vi "configuration UI.vi"() -> ()   [LabVIEW 2015, in "UI Reference editor node.lvclass"]
uses:
  UI Reference editor node.lvclass
  <vilib>/NI/Configuration Framework/Node/NodeRef.ctl
  <vilib>/NI/Configuration Framework/Node/NISE_CEF_Node.lvclass
  <vilib>/NI/AMC/Message Queue.ctl
  <vilib>/NI/AMC/Message.ctl
  <vilib>/NI/Tools/Keyed Array/KeyedArray.ctl
  <vilib>/NI/Configuration Framework/Node/UserEventRef.ctl
  <vilib>/NI/Configuration Framework/Controls/EventCluster.ctl
  <vilib>/NI/DCAF UI Toolkit/Controls/Configure.ctl
  <vilib>/NI/DCAF UI Toolkit/Controls/Add.ctl
  <vilib>/NI/DCAF UI Toolkit/Controls/Remove.ctl
  module/configuration/UI Reference configuration.lvclass
  <vilib>/Utility/miscctls.llb/LVPositionTypeDef.ctl
  <vilib>/NI/Module Execution Interface/Engine Configuration/engine configuration.lvclass
  <vilib>/NI/DCAF/Tag Editor Core/Configuration Editor/Classes/Engine Parent/Engine Parent Editor Node.lvclass
  <vilib>/NI/Tag Bus/tag/tag descriptor.lvclass
  <vilib>/NI/Tag Bus/tag/Data Type.ctl
  <vilib>/NI/Tag Bus/tag/tag descriptor.lvclass/tag descriptor.ctl
  module/configuration/UI Reference configuration.lvclass/UI Reference configuration.ctl
  UI Reference editor node.lvclass/UI Reference editor node.ctl
  <vilib>/NI/Tag Bus/tag/write tag name.vi
  <vilib>/NI/Tag Bus/tag/write data type.vi
  module/configuration/Read VI name.vi
  <vilib>/NI/DCAF/Tag Editor Core/Configuration Editor/Classes/Module editor node/Read Module Configuration.vi
  <vilib>/NI/Configuration Framework/serializable configuration/NISE_CEF_serializable configuration.lvclass
  <vilib>/NI/Tag Bus Module Framework/module configuration/TBM module configuration.lvclass
  <vilib>/NI/Configuration Framework/NISE_CEF_TreeControl.lvlib
  <vilib>/NI/DCAF/Tag Editor Core/Configuration Editor/Classes/Module editor node/module editor node.lvclass
  <vilib>/NI/DCAF UI Toolkit/Controls/DCAF UI Elements.lvlib
  <vilib>/NI/Tools/Keyed Array/Tools_KeyedArray.lvlib
  <vilib>/NI/AMC/AMC.lvlib
panel:
  in  "Top Level Tab Control":enum32{"UI Configuration"}(tab)
  in  "channel":i32(listbox)
  out "UI to Load":string
  in  "browse":bool
  in  "autogen":bool
  in  "Add Button":T1
  in  "Remove Button":T2
  in  "settings":T3
  in  "hidden_Add":bool
  in  "hidden_settings":bool
  in  "hidden_remove":bool
  in  "user event":T4
  in  "main queue":T5
  in  "node ref":T6
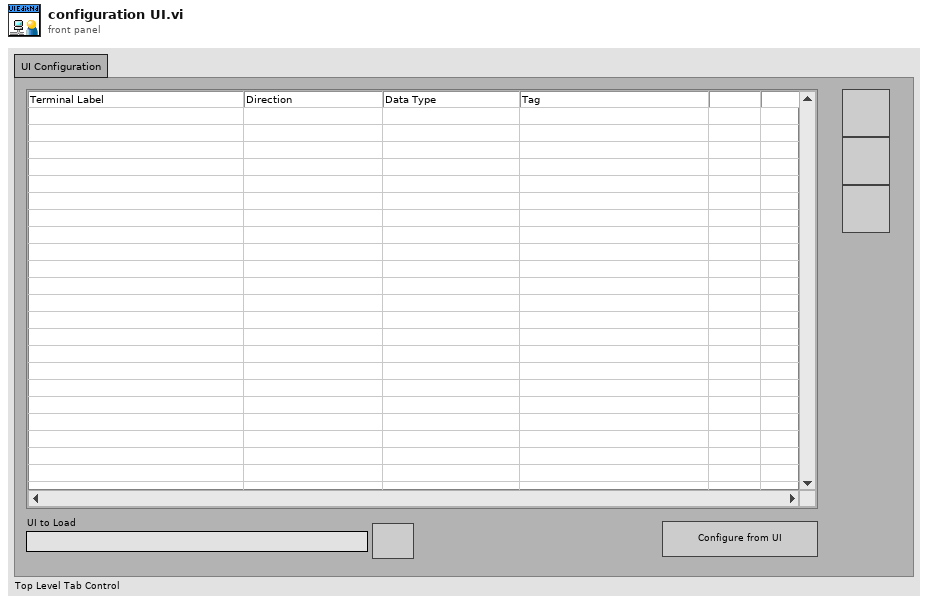
[diagram p1: front panel]
types:
  T1 = typedef "DCAF UI Elements.lvlib/Add.ctl" = bool
  T2 = typedef "DCAF UI Elements.lvlib/Remove.ctl" = bool
  T3 = typedef "DCAF UI Elements.lvlib/Configure.ctl" = bool
  T4 = typedef "NISE_CEF_Node.lvclass/UserEventRef.ctl" = refnum<user-event>
  T5 = typedef "AMC.lvlib/Message Queue.ctl" = refnum<queue>
  T6 = typedef "NISE_CEF_Node.lvclass/NodeRef.ctl" = refnum<data-value>
  T7 = typedef "LVPositionTypeDef.ctl" = cluster{"Left":i32, "Top":i32}
  T8 = typedef "NISE_CEF_TreeControl.lvlib/EventCluster.ctl" = cluster{"command":string, "data":string}
  T9 = typedef "tag bus.lvlib/tag descriptor.lvclass/Data Type.ctl" = enum16{"Double", "Single", "I64", "I32", "I16", "I8", "U64", "U32", "U16", "U8", "Boolean", "String", "Array of Double", "Array of Single", "Array of I64", "Array of I32", "Array of I16", "Array of I8", "Array of U64", "Array of U32", "Array of U16", "Array of U8", "Array of Boolean", "Array of String"}
  T10 = typedef "UI Reference editor node.lvclass/table line.ctl" = cluster{"channel":refnum<class "TBM channel.lvclass">, "tag name":string}
  T11 = typedef "LVPoint32TypeDef.ctl" = cluster{"Horizontal":i32, "Vertical":i32}
  T12 = typedef "LVRowAndColumnTypeDef.ctl" = cluster{"Row":i32, "Column":i32}
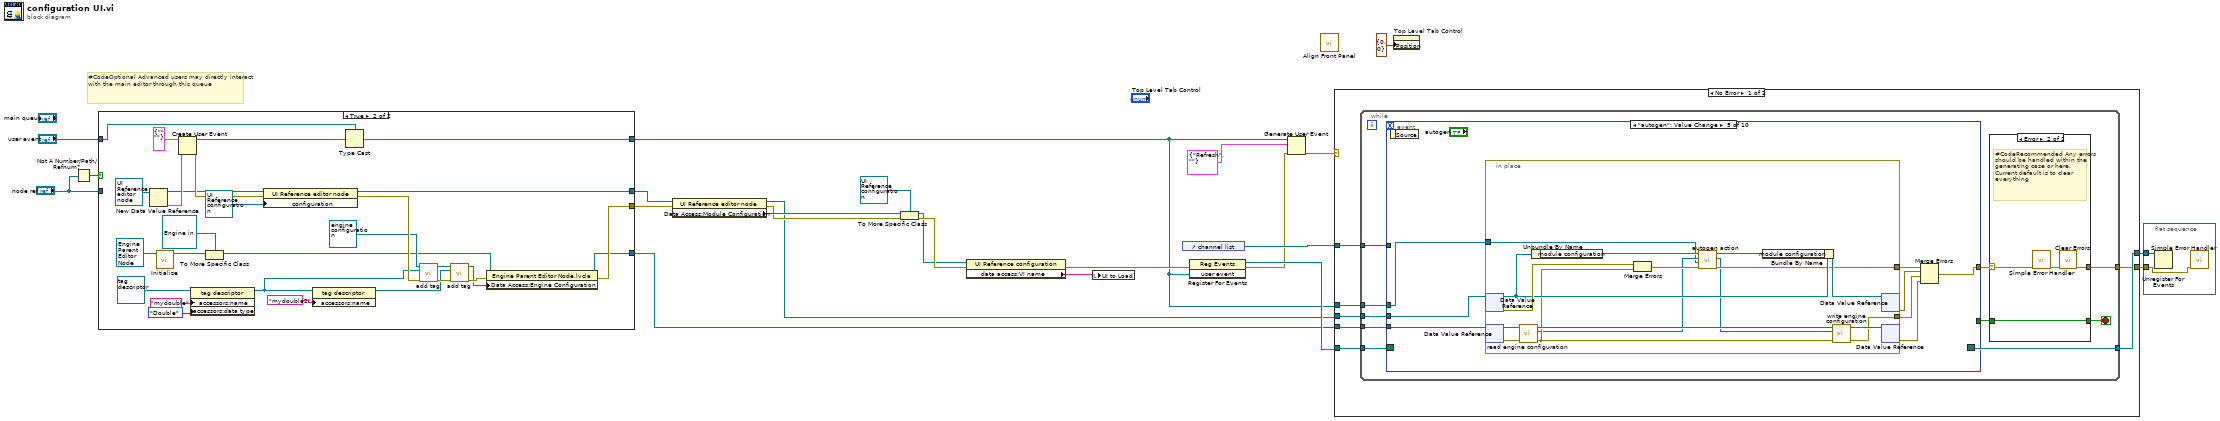
[diagram p0: block diagram]
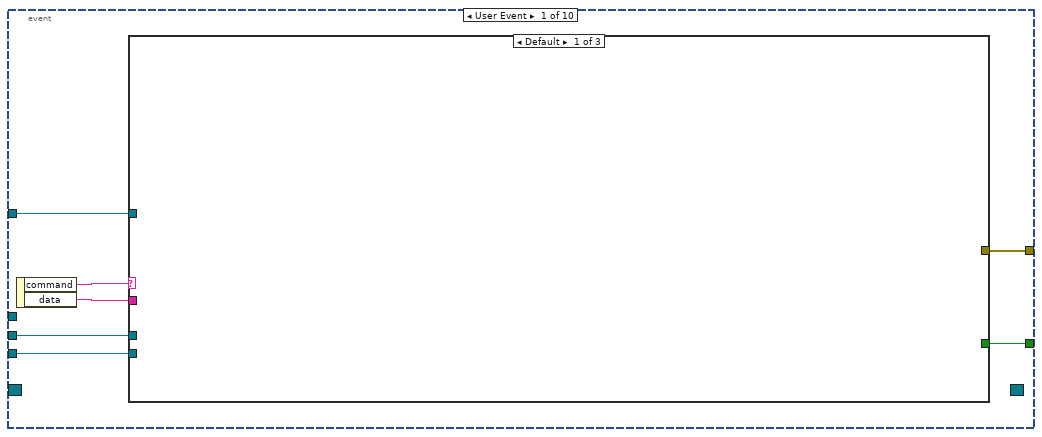
[diagram p3: hidden frame]
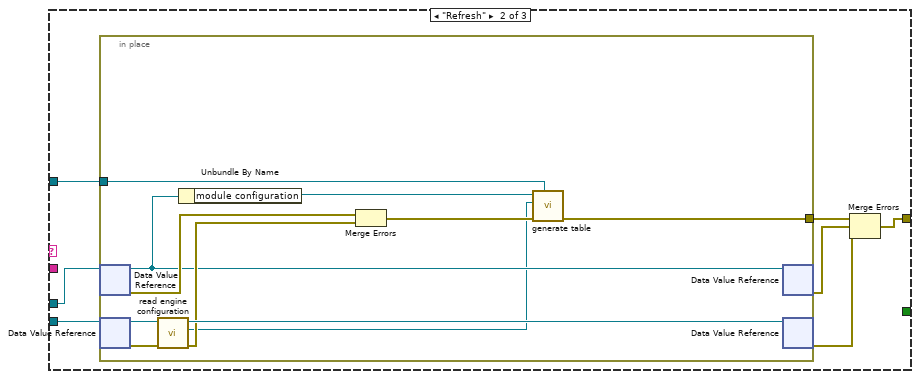
[diagram p4: hidden frame]
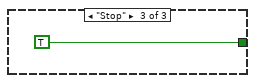
[diagram p5: hidden frame]
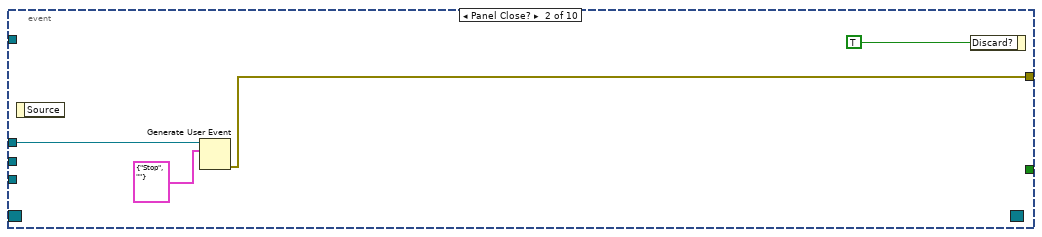
[diagram p6: hidden frame]
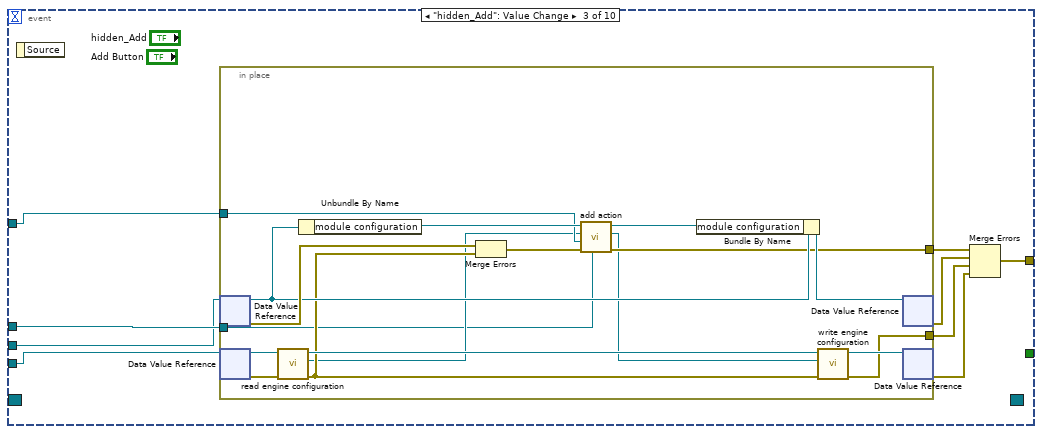
[diagram p7: hidden frame]
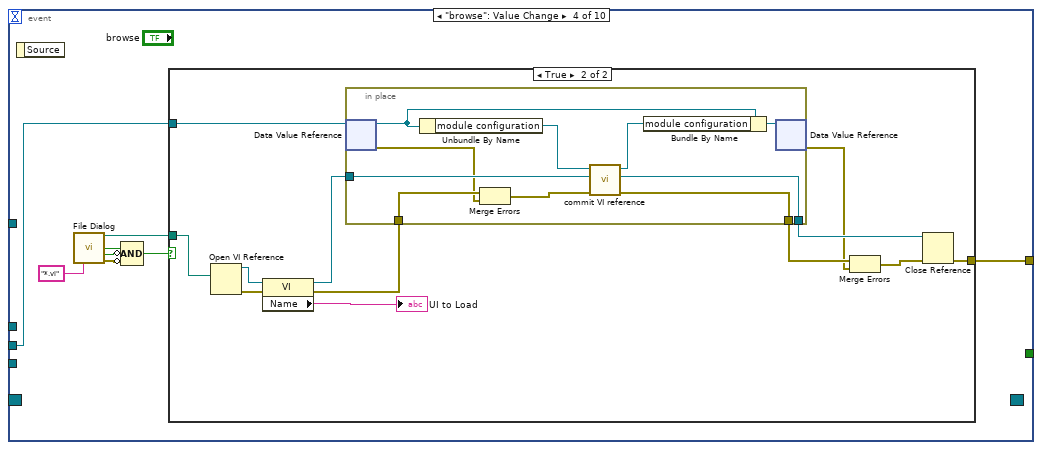
[diagram p8: hidden frame]
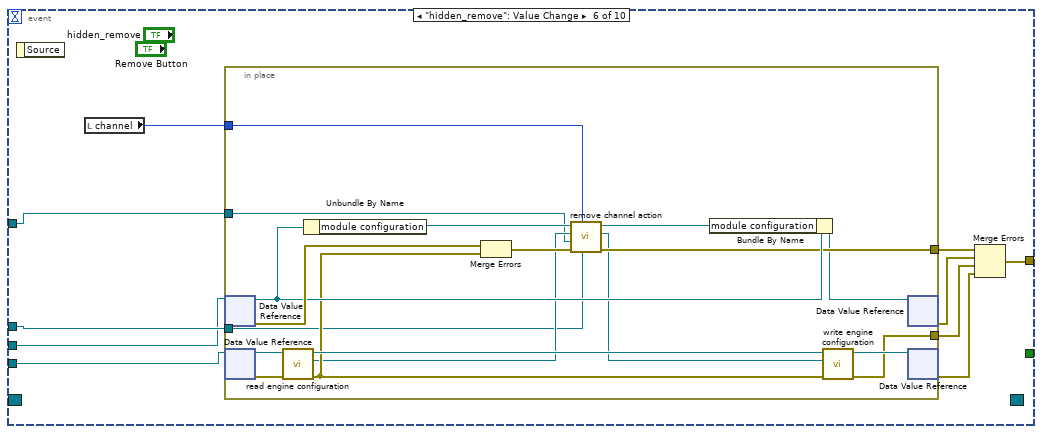
[diagram p10: hidden frame]
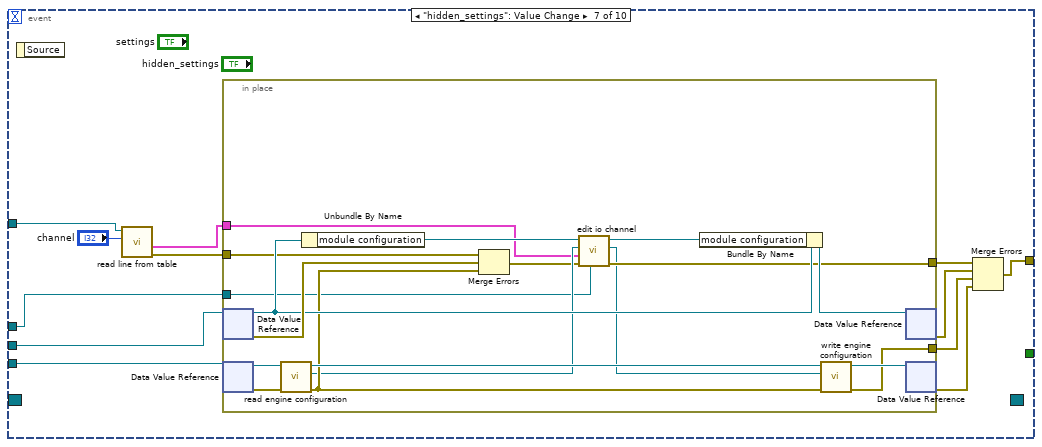
[diagram p11: hidden frame]
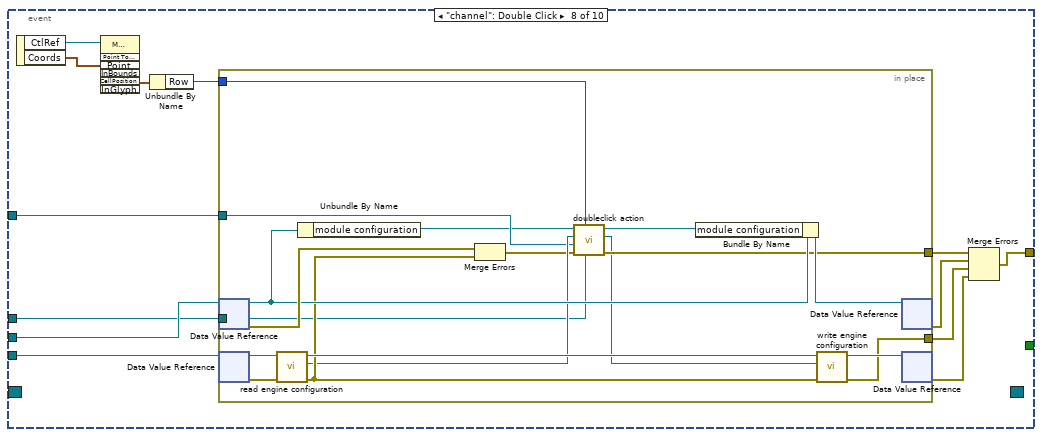
[diagram p12: hidden frame]
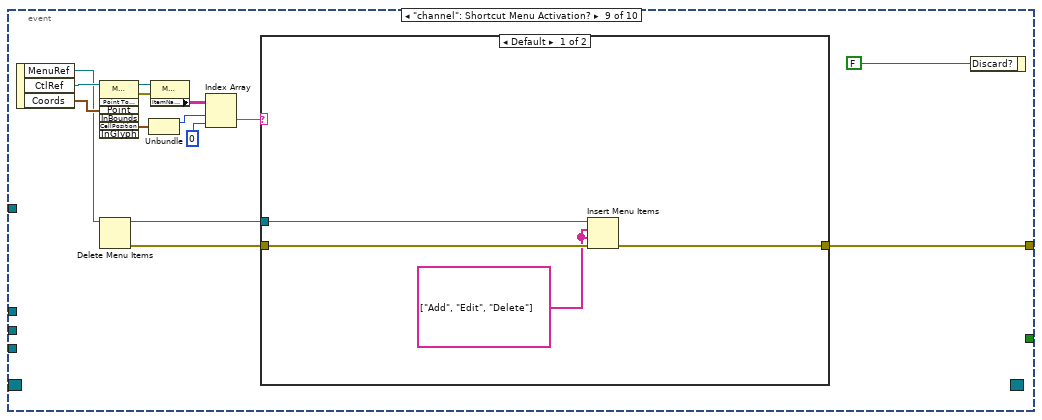
[diagram p13: hidden frame]
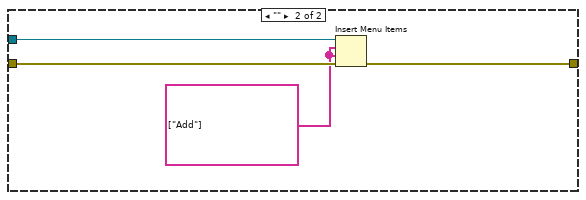
[diagram p14: hidden frame]
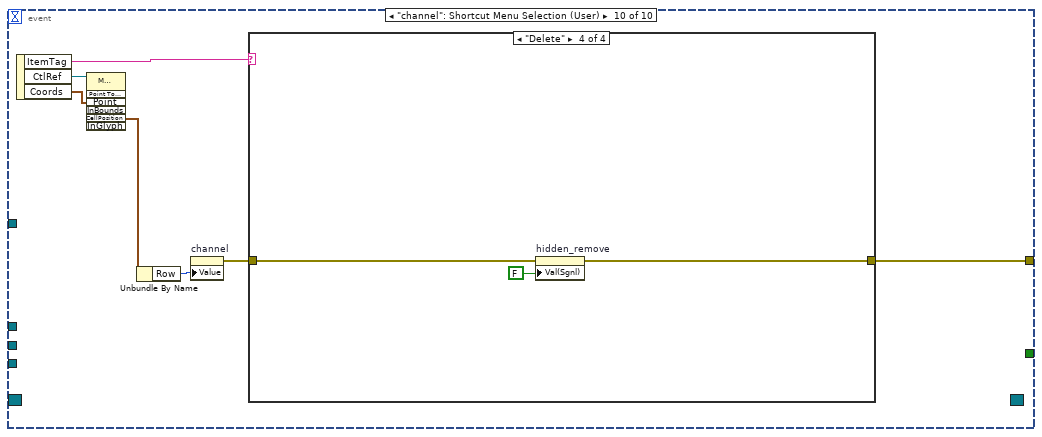
[diagram p15: hidden frame]
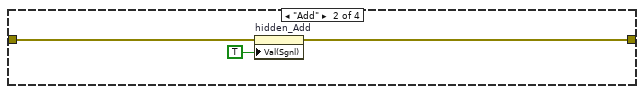
[diagram p17: hidden frame]
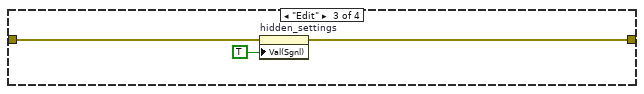
[diagram p18: hidden frame]
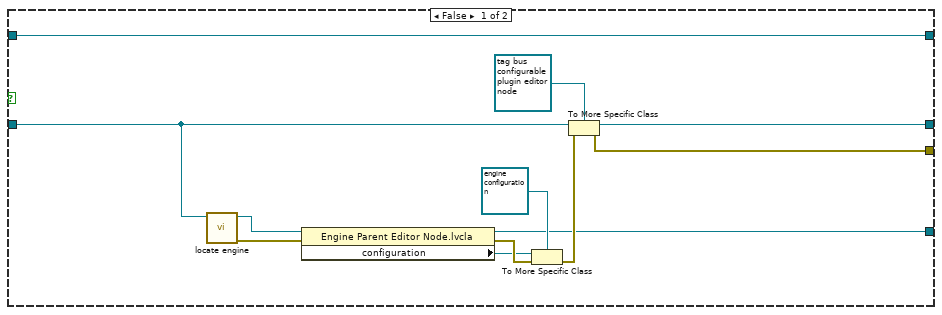
[diagram p20: hidden frame]
diagram:
  # "#CodeOptional Advanced users may directly interact with the main editor through this queue"
  n1 = Not A Number/Path/Refnum?(number/path/refnum="node ref") -> (NaN/Path/Refnum?=w17:bool)
  n2 = case shown="True" w17 {
    tunnel: "user event" -> [w35 w41]
    tunnel: [w35 w42] -> w5
    tunnel: "node ref" -> [w33 _]
    tunnel: [w32 w57] -> w12
    tunnel: [w31 w39] -> w15
    tunnel: [w24 w37] -> w10
    frame False {
      n3 = call <vilib>:"locate engine.vi"("component"=w33) -> ("error out"=w28:errorcluster, "engine"=w30:refnum<data-value>)  [unwired: 9 in]
      n4 = property class="Engine Parent Editor Node.lvcla"(reference=w30, error in=w28) -> (reference out=w24:refnum<data-value>, error out=w27:errorcluster, "configuration"=w26:refnum<class "NISE_CEF_serializable configuration.lvclass">)
      n5 = To More Specific Class(target class=refnum<class "engine configuration.lvclass"> refnum ("engine configuration.lvclass"), reference=w26, error in=w27) -> (error out=w25:errorcluster)  [unwired: 1 out]
      n6 = To More Specific Class(target class=refnum<data-value> refnum ("data value reference"), reference=w33, error in=w25) -> (specific class reference=w32:refnum<data-value>, error out=w31:errorcluster)
    }
    frame True {
      n7 = New Data Value Reference(data value=refnum<class "UI Reference editor node.lvclass"> refnum ("tag bus configurable plugin editor node")) -> (data value reference=w56:refnum<data-value>, error out=w59:errorcluster)  [unwired: 1 in]
      n8 = call-dynamic "Initialize.vi"("Engine in"=refnum<class "Engine Parent Editor Node.lvclass"> refnum) -> ("data value reference"=w55:T6)  [unwired: 8 in, 2 out]
      n9 = Create User Event(user event datatype=T8 {"command"="", "data"=""} ("event data"), error in=w59) -> (user event=w62:refnum<user-event>, error out=w58:errorcluster)
      n10 = property class="tag descriptor"(reference=refnum<class "tag descriptor.lvclass"> refnum ("tag descriptor"), "accessors:name"="mydouble" ("name"), "accessors:data type"=Data_Type."Double" ("data type")) -> (reference out=w43:refnum<class "tag descriptor.lvclass">)  [unwired: 1 in, 1 out]
      n11 = To More Specific Class(target class=refnum<data-value> refnum ("data value reference"), reference=w55) -> (specific class reference=w38:refnum<data-value>)  [unwired: 1 in, 1 out]
      n12 = property class="UI Reference editor node"(reference=w56, error in=w58, "configuration"=refnum<class "UI Reference configuration.lvclass"> refnum ("tag bus configurable plugin module configuration")) -> (reference out=w57:refnum<data-value>, error out=w49:errorcluster)
      n13 = property class="tag descriptor"(reference=w43, "accessors:name"="mydouble2" ("name")) -> (reference out=w44:refnum<class "tag descriptor.lvclass">)  [unwired: 1 in, 1 out]
      n14 = Type Cast(type=w41, x=w62) -> (*(type *) &x=w42:T4)
      n15 = call <vilib>:"add tag.vi"("error in"=w49, "tag descriptor"=w43, "engine configuration in"=refnum<class "engine configuration.lvclass"> refnum ("Engine Configuration")) -> ("error out"=w47:errorcluster, "engine configuration out"=w46:refnum<class "engine configuration.lvclass">)  [unwired: 7 in]
      n16 = call <vilib>:"add tag.vi"("error in"=w47, "tag descriptor"=w44, "engine configuration in"=w46) -> ("error out"=w45:errorcluster, "engine configuration out"=w36:refnum<class "engine configuration.lvclass">)  [unwired: 7 in]
      n17 = property class="Engine Parent Editor Node.lvcla"(reference=w38, error in=w45, "Data Access:Engine Configuration"=w36) -> (reference out=w37:refnum<data-value>, error out=w39:errorcluster)
    }
  }
  n18 = property class="UI Reference editor node"(reference=w12, error in=w15) -> (reference out=w11:refnum<data-value>, error out=w18:errorcluster, "Data Access:Module Configuration"=w19:refnum<class "TBM module configuration.lvclass">)
  n19 = To More Specific Class(target class=refnum<class "UI Reference configuration.lvclass"> refnum ("tag bus configurable plugin module configuration"), reference=w19, error in=w18) -> (specific class reference=w7:refnum<class "UI Reference configuration.lvclass">, error out=w13:errorcluster)
  n20 = property class="UI Reference configuration"(reference=w7, error in=w13) -> (error out=w8:errorcluster, "data access:VI name"=w6:string)  [unwired: 1 out]
  n21 = local write "UI to Load"(w6) -> ()
  n22 = control-ref of="channel list"() -> (w9:refnum<vi>)
  n23 = register-events(error in=w8, w5) -> (reference out=w23:refnum<event-registration>, error out=w3:errorcluster)  [unwired: 1 in]
  n24 = Generate User Event(user event=w5, event data cluster=T8 {"command"="Refresh", "data"=""} ("event data"), error in=w3) -> (error out=w2:errorcluster)  [unwired: 1 in, 1 out]
  n25 = call <vilib>:"Align Front Panel.vi"() -> ()  [unwired: 10 in, 2 out]
  n26 = case shown="No Error" w2 {
    selector: w2 -> [_ w325]
    tunnel: w23 -> [w70 w326]
    tunnel: [w69 w326] -> w22
    tunnel: [w68 w325] -> w21
    tunnel: w11 -> [w67 _]
    tunnel: w10 -> [w66 _]
    tunnel: w9 -> [w65 _]
    tunnel: w5 -> [w64 _]
    frame No Error {
      n27 = while {
        tunnel: w70 -> [w80]
        tunnel: [w79] -> w69
        tunnel: w67 -> [w75]
        tunnel: w66 -> [w74]
        tunnel: w64 -> [w73]
        tunnel: w65 -> [w71]
        tunnel: [w76] -> w68
        stop <- w78 stop-if-true
        n28 = event shown="[4] \"autogen\": Value Change" {
          selector: w80 -> [_ _ _ _ _ _ _ _ _ _]
          dyn-events: [_ _ _ _ _ _ _ _ _ _] -> w79
          timeout: _ -> [_ _ _ _ _ _ _ _ _ _]
          tunnel: [w93 _ _ _ _ _ _ _ _ _] -> w77
          tunnel: [w88 w113 w121 w144 w176 w202 w230 w260 w286 w311] -> w72
          tunnel: w75 -> [w91 _ w117 w143 w174 w197 w228 w258 _ _]
          tunnel: w74 -> [w90 _ w120 _ w175 w198 w229 w259 _ _]
          tunnel: w73 -> [_ w114 w118 _ w173 w200 w226 w257 _ _]
          tunnel: w71 -> [w87 _ w119 _ _ w199 w235 w256 _ _]
          event User Event {
            n29 = event-data() -> ("command"=w92:string, "data"=w89:string)  [unwired: 1 in]
            n30 = case shown="Default" w92 {
              tunnel: [_ _ TRUE] -> w93
              tunnel: w91 -> [_ w96 _]
              tunnel: w90 -> [_ w97 _]
              tunnel: w89 -> [_ _ _]
              tunnel: [_ w98 _] -> w88
              tunnel: w87 -> [_ w99 _]
              frame Default {
              }
              frame "Refresh" {
                n31 = in-place {
                  in-place-border: [w111] -> w100
                  in-place-border: w99 -> [w110]
                  n32 = in-place-dvr #1(w96) -> (w103:refnum<class "UI Reference editor node.lvclass">, w104:errorcluster)
                  n33 = in-place-dvr #2(w97) -> (w108:refnum<class "Engine Parent Editor Node.lvclass">, w107:errorcluster)
                  n34 = call <vilib>:"read engine configuration.vi"("error in"=w107, "Engine Parent Editor Node in"=w108) -> ("error out"=w105:errorcluster, "engine configuration"=w101:refnum<class "engine configuration.lvclass">, "Engine Parent Editor Node out"=w106:refnum<class "Engine Parent Editor Node.lvclass">)  [unwired: 7 in]
                  n35 = Unbundle By Name(w103) -> ("module configuration"=w102:refnum<class "UI Reference configuration.lvclass">)
                  n36 = Merge Errors(w104, w105) -> (w109:errorcluster)
                  n37 = call "generate table.vi"("table"=w110, "error in"=w109, "engine configuration"=w101, "tag bus configurable plugin module configuration"=w102) -> ("error out"=w111:errorcluster)  [unwired: 7 in]
                  n38 = in-place-dvr #1(w103) -> (w94:errorcluster)  [unwired: 1 out]
                  n39 = in-place-dvr #2(w106) -> (w95:errorcluster)  [unwired: 1 out]
                }
                n40 = Merge Errors(w100, w94, w95) -> (w98:errorcluster)
              }
              frame "Stop" {
              }
            }
          }
          event Panel Close? {
            n41 = event-data() -> ()  [unwired: 1 in, 1 out]
            n42 = Generate User Event(user event=w114, event data cluster=T8 {"command"="Stop", "data"=""} ("event data")) -> (error out=w113:errorcluster)  [unwired: 2 in, 1 out]
            n43 = event-data("Discard?"=TRUE) -> ()  [unwired: 1 in, 1 out]
          }
          event "hidden_Add": Value Change {
            n44 = event-data() -> ()  [unwired: 1 in, 1 out]
            n45 = in-place {
              in-place-border: [w133] -> w122
              in-place-border: [w136] -> w125
              in-place-border: w119 -> [w128]
              in-place-border: w118 -> [w126]
              n46 = in-place-dvr #3(w117) -> (w139:refnum<class "UI Reference editor node.lvclass">, w140:errorcluster)
              n47 = in-place-dvr #4(w120) -> (w142:refnum<class "Engine Parent Editor Node.lvclass">, w141:errorcluster)
              n48 = call <vilib>:"read engine configuration.vi"("error in"=w141, "Engine Parent Editor Node in"=w142) -> ("error out"=w135:errorcluster, "engine configuration"=w127:refnum<class "engine configuration.lvclass">, "Engine Parent Editor Node out"=w138:refnum<class "Engine Parent Editor Node.lvclass">)  [unwired: 7 in]
              n49 = Unbundle By Name(w139) -> ("module configuration"=w129:refnum<class "UI Reference configuration.lvclass">)
              n50 = Merge Errors(w140, w135) -> (w132:errorcluster)
              n51 = call "add action.vi"("user event"=w126, "error in"=w132, "channel list"=w128, "engine configuration in"=w127, "UI Reference configuration in"=w129) -> ("error out"=w133:errorcluster, "engine configuration out"=w130:refnum<class "engine configuration.lvclass">, "UI Reference configuration out"=w131:refnum<class "UI Reference configuration.lvclass">)  [unwired: 4 in]
              n52 = Bundle By Name(cluster=w139, "module configuration"=w131) -> (w134:refnum<class "UI Reference editor node.lvclass">)
              n53 = call <vilib>:"write engine configuration.vi"("error in"=w135, "engine configuration"=w130, "Engine Parent Editor Node in"=w138) -> ("error out"=w136:errorcluster, "Engine Parent Editor Node out"=w137:refnum<class "Engine Parent Editor Node.lvclass">)  [unwired: 7 in]
              n54 = in-place-dvr #3(w134) -> (w124:errorcluster)  [unwired: 1 out]
              n55 = in-place-dvr #4(w137) -> (w123:errorcluster)  [unwired: 1 out]
            }
            n56 = Merge Errors(w122, w124, w125, w123) -> (w121:errorcluster)
          }
          event "browse": Value Change {
            n57 = event-data() -> ()  [unwired: 1 in, 1 out]
            n58 = call "File Dialog"("pattern (all files)"="*.vi") -> ("selected path"=w145:path, "exists"=w149:bool, "cancelled"=w148:bool, "error out"=w147:errorcluster)  [unwired: 11 in]
            n59 = Compound Arithmetic op=AND(w149, invert w148, invert w147) -> (w146:bool)
            n60 = case shown="True" w146 {
              tunnel: w145 -> [_ w162]
              tunnel: [_ w158] -> w144
              tunnel: w143 -> [_ w153]
              frame False {
              }
              frame True {
                n61 = Open VI Reference(vi path=w162) -> (vi reference=w160:refnum<vi>, error out=w161:errorcluster)  [unwired: 5 in]
                n62 = property class="VI"(reference=w160, error in=w161) -> (reference out=w155:refnum<vi>, error out=w156:errorcluster, "Name"=→"UI to Load":string)
                n63 = in-place {
                  in-place-border: [w172] -> w157
                  in-place-border: w156 -> [w171]
                  in-place-border: w155 -> [w170]
                  in-place-border: [w169] -> w154
                  n64 = in-place-dvr #5(w153) -> (w166:refnum<class "UI Reference editor node.lvclass">, w163:errorcluster)
                  n65 = Unbundle By Name(w166) -> ("module configuration"=w168:refnum<class "UI Reference configuration.lvclass">)
                  n66 = Merge Errors(w171, w163) -> (w164:errorcluster)
                  n67 = call "commit VI reference.vi"("error in"=w164, "VI Refnum in"=w170, "UI Reference configuration in"=w168) -> ("error out"=w169:errorcluster, "VI Refnum out"=w172:refnum<vi>, "UI Reference configuration out"=w165:refnum<class "UI Reference configuration.lvclass">)  [unwired: 6 in]
                  n68 = Bundle By Name(cluster=w166, "module configuration"=w165) -> (w167:refnum<class "UI Reference editor node.lvclass">)
                  n69 = in-place-dvr #5(w167) -> (w151:errorcluster)  [unwired: 1 out]
                }
                n70 = Merge Errors(w154, w151) -> (w152:errorcluster)
                n71 = Close Reference(reference=w157, error in (no error)=w152) -> (error out=w158:errorcluster)
              }
            }
          }
          event "autogen": Value Change {
            n72 = event-data() -> ()  [unwired: 1 in, 1 out]
            n73 = in-place {
              in-place-border: [w187] -> w177
              in-place-border: [w190] -> w180
              in-place-border: w173 -> [w181]
              n74 = in-place-dvr #6(w174) -> (w193:refnum<class "UI Reference editor node.lvclass">, w194:errorcluster)
              n75 = in-place-dvr #7(w175) -> (w196:refnum<class "Engine Parent Editor Node.lvclass">, w195:errorcluster)
              n76 = call <vilib>:"read engine configuration.vi"("error in"=w195, "Engine Parent Editor Node in"=w196) -> ("error out"=w189:errorcluster, "engine configuration"=w185:refnum<class "engine configuration.lvclass">, "Engine Parent Editor Node out"=w192:refnum<class "Engine Parent Editor Node.lvclass">)  [unwired: 7 in]
              n77 = Unbundle By Name(w193) -> ("module configuration"=w184:refnum<class "UI Reference configuration.lvclass">)
              n78 = Merge Errors(w194, w189) -> (w186:errorcluster)
              n79 = call "autogen action.vi"("error in"=w186, "user event"=w181, "engine configuration in"=w185, "UI Reference configuration in"=w184) -> ("error out"=w187:errorcluster, "engine configuration out"=w182:refnum<class "engine configuration.lvclass">, "UI Reference configuration out"=w183:refnum<class "UI Reference configuration.lvclass">)  [unwired: 5 in]
              n80 = Bundle By Name(cluster=w193, "module configuration"=w183) -> (w188:refnum<class "UI Reference editor node.lvclass">)
              n81 = call <vilib>:"write engine configuration.vi"("error in"=w189, "engine configuration"=w182, "Engine Parent Editor Node in"=w192) -> ("error out"=w190:errorcluster, "Engine Parent Editor Node out"=w191:refnum<class "Engine Parent Editor Node.lvclass">)  [unwired: 7 in]
              n82 = in-place-dvr #6(w188) -> (w179:errorcluster)  [unwired: 1 out]
              n83 = in-place-dvr #7(w191) -> (w178:errorcluster)  [unwired: 1 out]
            }
            n84 = Merge Errors(w177, w179, w180, w178) -> (w176:errorcluster)
          }
          event "hidden_remove": Value Change {
            n85 = event-data() -> ()  [unwired: 1 in, 1 out]
            n86 = local read "channel"() -> (w201:i32)
            n87 = in-place {
              in-place-border: [w216] -> w203
              in-place-border: [w218] -> w206
              in-place-border: w201 -> [w211]
              in-place-border: w200 -> [w210]
              in-place-border: w199 -> [w209]
              n88 = in-place-dvr #8(w197) -> (w221:refnum<class "UI Reference editor node.lvclass">, w222:errorcluster)
              n89 = in-place-dvr #9(w198) -> (w224:refnum<class "Engine Parent Editor Node.lvclass">, w223:errorcluster)
              n90 = call <vilib>:"read engine configuration.vi"("error in"=w223, "Engine Parent Editor Node in"=w224) -> ("error out"=w217:errorcluster, "engine configuration"=w214:refnum<class "engine configuration.lvclass">, "Engine Parent Editor Node out"=w220:refnum<class "Engine Parent Editor Node.lvclass">)  [unwired: 7 in]
              n91 = Unbundle By Name(w221) -> ("module configuration"=w212:refnum<class "UI Reference configuration.lvclass">)
              n92 = Merge Errors(w222, w217) -> (w215:errorcluster)
              n93 = call "remove channel action.vi"("user event"=w210, "channel"=w211, "error in"=w215, "channel list"=w209, "engine configuration in"=w214, "UI Reference configuration in"=w212) -> ("error out"=w216:errorcluster, "engine configuration out"=w213:refnum<class "engine configuration.lvclass">, "UI Reference configuration out"=w207:refnum<class "UI Reference configuration.lvclass">)  [unwired: 3 in]
              n94 = Bundle By Name(cluster=w221, "module configuration"=w207) -> (w208:refnum<class "UI Reference editor node.lvclass">)
              n95 = call <vilib>:"write engine configuration.vi"("error in"=w217, "engine configuration"=w213, "Engine Parent Editor Node in"=w220) -> ("error out"=w218:errorcluster, "Engine Parent Editor Node out"=w219:refnum<class "Engine Parent Editor Node.lvclass">)  [unwired: 7 in]
              n96 = in-place-dvr #8(w208) -> (w205:errorcluster)  [unwired: 1 out]
              n97 = in-place-dvr #9(w219) -> (w204:errorcluster)  [unwired: 1 out]
            }
            n98 = Merge Errors(w203, w205, w206, w204) -> (w202:errorcluster)
          }
          event "hidden_settings": Value Change {
            n99 = event-data() -> ()  [unwired: 1 in, 1 out]
            n100 = call "read line from table.vi"("line number"="channel", "channels table"=w235) -> ("error out"=w227:errorcluster, "line"=w225:T10)  [unwired: 6 in, 2 out]
            n101 = in-place {
              in-place-border: [w244] -> w231
              in-place-border: [w248] -> w234
              in-place-border: w227 -> [w245]
              in-place-border: w226 -> [w238]
              in-place-border: w225 -> [w237]
              n102 = in-place-dvr #10(w228) -> (w251:refnum<class "UI Reference editor node.lvclass">, w252:errorcluster)
              n103 = in-place-dvr #11(w229) -> (w254:refnum<class "Engine Parent Editor Node.lvclass">, w253:errorcluster)
              n104 = call <vilib>:"read engine configuration.vi"("error in"=w253, "Engine Parent Editor Node in"=w254) -> ("error out"=w247:errorcluster, "engine configuration"=w240:refnum<class "engine configuration.lvclass">, "Engine Parent Editor Node out"=w250:refnum<class "Engine Parent Editor Node.lvclass">)  [unwired: 7 in]
              n105 = Unbundle By Name(w251) -> ("module configuration"=w241:refnum<class "UI Reference configuration.lvclass">)
              n106 = Merge Errors(w245, w252, w247) -> (w239:errorcluster)
              n107 = call "edit io channel.vi"("user event"=w238, "error in"=w239, "line"=w237, "engine configuration in"=w240, "tag bus configurable plugin module configuration in"=w241) -> ("error out"=w244:errorcluster, "engine configuration"=w242:refnum<class "engine configuration.lvclass">, "tag bus configurable plugin module configuration out"=w243:refnum<class "UI Reference configuration.lvclass">)  [unwired: 4 in]
              n108 = Bundle By Name(cluster=w251, "module configuration"=w243) -> (w246:refnum<class "UI Reference editor node.lvclass">)
              n109 = call <vilib>:"write engine configuration.vi"("error in"=w247, "engine configuration"=w242, "Engine Parent Editor Node in"=w250) -> ("error out"=w248:errorcluster, "Engine Parent Editor Node out"=w249:refnum<class "Engine Parent Editor Node.lvclass">)  [unwired: 7 in]
              n110 = in-place-dvr #10(w246) -> (w233:errorcluster)  [unwired: 1 out]
              n111 = in-place-dvr #11(w249) -> (w232:errorcluster)  [unwired: 1 out]
            }
            n112 = Merge Errors(w231, w233, w234, w232) -> (w230:errorcluster)
          }
          event "channel": Double Click {
            n113 = event-data() -> ("CtlRef"=w267:refnum<vi>, "Coords"=w266:T11)  [unwired: 1 in]
            n114 = invoke class="MCListbox (strict)" method="Point To Row Column"(reference=w267, "Point"=w266) -> ("CellPosition"=w265:T12)  [unwired: 5 in, 6 out]
            n115 = Unbundle By Name(w265) -> ("Row"=w255:i32)
            n116 = in-place {
              in-place-border: [w276] -> w261
              in-place-border: [w279] -> w264
              in-place-border: w257 -> [w272]
              in-place-border: w256 -> [w271]
              in-place-border: w255 -> [w269]
              n117 = in-place-dvr #12(w258) -> (w282:refnum<class "UI Reference editor node.lvclass">, w283:errorcluster)
              n118 = in-place-dvr #13(w259) -> (w285:refnum<class "Engine Parent Editor Node.lvclass">, w284:errorcluster)
              n119 = call <vilib>:"read engine configuration.vi"("error in"=w284, "Engine Parent Editor Node in"=w285) -> ("error out"=w278:errorcluster, "engine configuration"=w273:refnum<class "engine configuration.lvclass">, "Engine Parent Editor Node out"=w281:refnum<class "Engine Parent Editor Node.lvclass">)  [unwired: 7 in]
              n120 = Unbundle By Name(w282) -> ("module configuration"=w270:refnum<class "UI Reference configuration.lvclass">)
              n121 = Merge Errors(w283, w278) -> (w268:errorcluster)
              n122 = call "doubleclick action.vi"("user event"=w272, "Row"=w269, "error in"=w268, "channel list"=w271, "engine configuration in"=w273, "UI Reference configuration in"=w270) -> ("error out"=w276:errorcluster, "engine configuration out"=w274:refnum<class "engine configuration.lvclass">, "UI Reference configuration out"=w275:refnum<class "UI Reference configuration.lvclass">)  [unwired: 3 in]
              n123 = Bundle By Name(cluster=w282, "module configuration"=w275) -> (w277:refnum<class "UI Reference editor node.lvclass">)
              n124 = call <vilib>:"write engine configuration.vi"("error in"=w278, "engine configuration"=w274, "Engine Parent Editor Node in"=w281) -> ("error out"=w279:errorcluster, "Engine Parent Editor Node out"=w280:refnum<class "Engine Parent Editor Node.lvclass">)  [unwired: 7 in]
              n125 = in-place-dvr #12(w277) -> (w263:errorcluster)  [unwired: 1 out]
              n126 = in-place-dvr #13(w280) -> (w262:errorcluster)  [unwired: 1 out]
            }
            n127 = Merge Errors(w261, w263, w264, w262) -> (w260:errorcluster)
          }
          event "channel": Shortcut Menu Activation? {
            n128 = event-data() -> ("MenuRef"=w296:refnum<k9>, "CtlRef"=w298:refnum<vi>, "Coords"=w297:T11)  [unwired: 1 in]
            n129 = invoke class="MCListbox (strict)" method="Point To Row Column"(reference=w298, "Point"=w297) -> (reference out=w295:refnum<vi>, error out=w294:errorcluster, "CellPosition"=w293:T12)  [unwired: 5 in, 4 out]
            n130 = Delete Menu Items(9:w296) -> (0:w287:errorcluster, 3:w288:refnum<k9>)  [unwired: 3 in]
            n131 = Unbundle(w293) -> ("Row"=w291:i32)  [unwired: 1 out]
            n132 = property class="MCListbox (strict)"(reference=w295, error in=w294) -> ("ItemNames"=w292:string[][])  [unwired: 2 out]
            n133 = Index Array(array=w292, index (row)=w291, index (col)=0 ("disabled index (col)")) -> (element=w289:string)
            n134 = case shown="Default" w289 {
              tunnel: w288 -> [w303 w307]
              tunnel: w287 -> [w302 w306]
              tunnel: [w301 w305] -> w286
              frame Default {
                w300 = string[] ["Add", "Edit", "Delete"] ("item names")
                n135 = Insert Menu Items(6:w302, 7:w300, 8:w300, 9:w303) -> (0:w301:errorcluster)  [unwired: 2 in, 2 out]
              }
              frame "" {
                w304 = string[] ["Add"] ("item names")
                n136 = Insert Menu Items(6:w306, 7:w304, 8:w304, 9:w307) -> (0:w305:errorcluster)  [unwired: 2 in, 2 out]
              }
            }
            n137 = event-data("Discard?"=FALSE) -> ()  [unwired: 1 in, 1 out]
          }
          event "channel": Shortcut Menu Selection (User) {
            n138 = event-data() -> ("ItemTag"=w312:string, "CtlRef"=w313:refnum<vi>, "Coords"=w314:T11)  [unwired: 1 in]
            n139 = invoke class="MCListbox (strict)" method="Point To Row Column"(reference=w313, "Point"=w314) -> ("CellPosition"=w309:T12)  [unwired: 5 in, 6 out]
            n140 = Unbundle By Name(w309) -> ("Row"=w308:i32)
            n141 = property on="channel" class="MCListbox (strict)"("Value"=w308) -> (error out=w310:errorcluster)  [unwired: 2 in, 1 out]
            n142 = case shown="\"Delete\"" w312 {
              tunnel: w310 -> [w315 w317 w321 w324]
              tunnel: [w315 w316 w320 w323] -> w311
              frame Default {
              }
              frame "Add" {
                n143 = property on="hidden_Add" class="Bool (strict)"(error in=w317, "Val(Sgnl)"=TRUE ("Value (Signaling)")) -> (error out=w316:errorcluster)  [unwired: 1 in, 1 out]
              }
              frame "Edit" {
                n144 = property on="hidden_settings" class="Bool (strict)"(error in=w321, "Val(Sgnl)"=TRUE ("Value (Signaling)")) -> (error out=w320:errorcluster)  [unwired: 1 in, 1 out]
              }
              frame "Delete" {
                n145 = property on="hidden_remove" class="Bool (strict)"(error in=w324, "Val(Sgnl)"=FALSE ("Value (Signaling)")) -> (error out=w323:errorcluster)  [unwired: 1 in, 1 out]
              }
            }
          }
        }
        n146 = case shown="Error" w72 {
          selector: w72 -> [w81 w85]
          tunnel: [w82 w86] -> w78
          tunnel: w77 -> [w82 w86]
          tunnel: [w81 w83] -> w76
          frame No Error {
          }
          frame Error {
            # "#CodeRecommended Any errors should be handled within the generating case or here. Current default is to clear everything"
            n147 = call <vilib>:"Simple Error Handler.vi"("error in (no error)"=w85) -> ("error out"=w84:errorcluster)  [unwired: 4 in, 4 out]
            n148 = call <vilib>:"Clear Errors.vi"("error in (no error)"=w84) -> ("error out"=w83:errorcluster)  [unwired: 5 in, 1 out]
          }
        }
      }
    }
    frame Error {
    }
  }
  n149 = property on="Top Level Tab Control" class="TabCtl (strict)"("Position"=T7 {"Left"=0, "Top"=0}) -> ()  [unwired: 2 in, 2 out]
  n150 = flat-sequence {
    tunnel: w22 -> [w328]
    tunnel: w21 -> [w327]
    frame #0 {
      n151 = Unregister For Events(event registration refnum=w328) -> ()  [unwired: 1 in, 1 out]
      n152 = call <vilib>:"Simple Error Handler.vi"("error in (no error)"=w327) -> ()  [unwired: 4 in, 5 out]
    }
  }
